vi "Read-Write Camera Settings to File.vi"(6 "Read(f)Write(t)":bool, 7 "Cam ID":u8, 8 "Error":errorcluster, 11 "Cam Setings":T1 {"Saturation" min=0 max=100 step=1; "Sharpness" min=0 max=100 step=1; "Brightness" min=0 max=100 step=1; "Exposure (%)" min=0.0 max=100.0 step=1.0}) -> (0 "Error Out":errorcluster, 3 "Cam Setings Out":T1 {"Saturation" min=0 max=100 step=1; "Sharpness" min=0 max=100 step=1; "Brightness" min=0 max=100 step=1; "Exposure (%)" min=0.0 max=100.0 step=1.0}, 5 "Found? Out":bool)   [LabVIEW 2017, in "VisionSystem.lvlib"]
uses:
  VisionSystem.lvlib
  TypeDefs/Cluster_Camera Settings.ctl
  <vilib>/Rock Robotics/WPI/Camera/WPI_CameraImageSize.ctl
  <vilib>/Rock Robotics/WPI/Camera/WPI_CameraFrameRate.ctl
  <vilib>/Rock Robotics/WPI/Camera/WPI_CameraWhite Balance Values.ctl
  <vilib>/Rock Robotics/WPI/Camera/WPI_CameraExposure Values.ctl
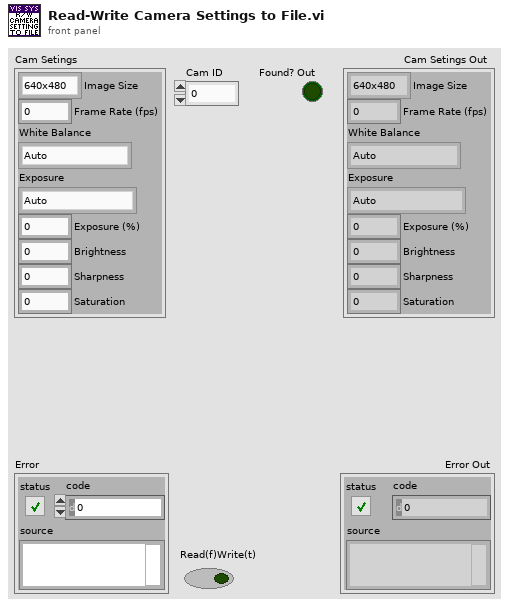
[diagram p1: front panel]
types:
  T1 = typedef "Cluster_Camera Settings.ctl" = cluster{"Image Size":T2, "Frame Rate (fps)":T3, "White Balance":T4, "Exposure":T5, "Exposure (%)":dbl, "Brightness":i32, "Sharpness":i32, "Saturation":i32}
  T2 = typedef "WPI_CameraImageSize.ctl" = enum16{"640x480", "320x240", "160x120", "Custom"}
  T3 = typedef "WPI_CameraFrameRate.ctl" = u32
  T4 = typedef "WPI_CameraWhite Balance Values.ctl" = enum16{"Auto", "Fixed indoor", "Fixed outdoor 1", "Fixed outdoor 2", "Fixed fluorescent 1", "Fixed fluorescent 2", "Hold current", "Custom"}
  T5 = typedef "WPI_CameraExposure Values.ctl" = enum16{"Auto", "Flicker-free 50 Hz", "Flicker-free 60 Hz", "Hold current", "Custom"}
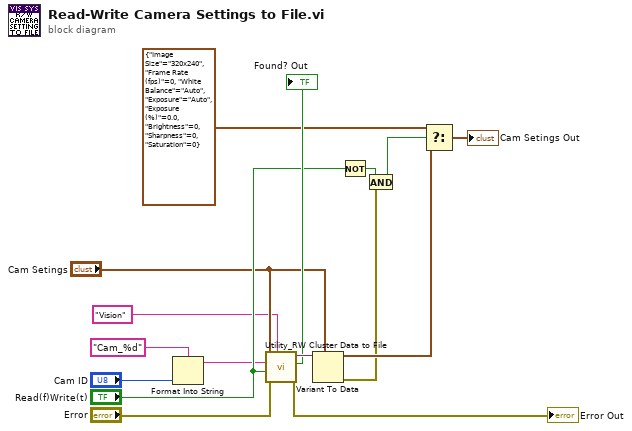
[diagram p0: block diagram]
diagram:
  n1 = Format Into String(format string="Cam_%d", "Cam ID") -> (resulting string=w6:string)  [unwired: 2 in, 1 out]
  n2 = call "Utility_RW Cluster Data to File.vi"("System"="Vision", "Error"="Error", "Read(f)Write(t)"="Read(f)Write(t)", "Data Name"=w6, "Cluster Data"="Cam Setings") -> ("Error Out"=→"Error Out":errorcluster, "Found? Out"=→"Found? Out":bool, "Cluster Data Out"=w13:variant)  [unwired: 4 in]
  n3 = Variant To Data(type="Cam Setings", Variant=w13) -> (data=w12:T1, error out=w7:errorcluster)  [unwired: 1 in]
  n4 = Not(x="Read(f)Write(t)") -> (.not. x?=w9:bool)
  n5 = And(x=w9, y=w7) -> (x .and. y?=w8:bool)
  n6 = Select(t=T1 {"Image Size"=enum."320x240", "Frame Rate (fps)"=0, "White Balance"=enum."Auto", "Exposure"=enum."Auto", "Exposure (%)"=0.0, "Brightness"=0, "Sharpness"=0, "Saturation"=0} ("Cam Setings"), s=w8, f=w12) -> (s? t:f=→"Cam Setings Out":T1)
